vi "Test App Process Error Handler is Used if Configured.vi"(8 "error in (no error)":errorcluster, 11 "Rig Test In":refnum<class "Application Test.lvclass">) -> (0 "error out":errorcluster, 3 "Rig Test Out":refnum<class "Application Test.lvclass">)   [LabVIEW 2020, in "Application Test.lvclass"]
uses:
  Application Test.lvclass
  C:/Program Files (x86)/National Instruments/LabVIEW 2020/vi.lib/Asteme/LUnit/Test Case.lvclass
  Mock Process/Mock Process.lvclass
  C:/Users/anton/Documents/GitHub/Triarc-Framework/source/Framework/Process/Process.lvclass
  Mock Error Handler/Mock Error Handler.lvclass
  C:/Users/anton/Documents/GitHub/Triarc-Framework/source/Framework/Error Handler Interface/Error Handler Interface.lvclass
  Framework/Process/Process.lvclass/Process.ctl
  Framework/Application/Application.lvclass/Application.ctl
  <vilib>/Asteme/LUnit/Test Case.lvclass/Test Case.ctl
  <vilib>/Asteme/LUnit/LUnit Assertion Result.lvclass/LUnit Assertion Result.ctl
  Framework/Process/Protected/Messaging/Enqueue Message.vi
  Framework/Process/Public/Lifecycle/Get Lifecycle State.vi
  Framework/Application/Private/Add Process to Map.vi
  Framework/Process/Protected/SubVIs/Set Context.vi
  Framework/Process/Protected/Messaging/Request Message.vi
  <vilib>/Asteme/LUnit/Palette/Pass.vi
  <vilib>/Asteme/LUnit/Palette/Fail.vi
  <vilib>/Asteme/LUnit/Variant to string.vi
  <vilib>/Asteme/LUnit/Set Assertion Type.vi
  Framework/Process/Private/SubVIs/Wait for finish.vi
  Framework/Process/Private/SubVIs/Set Lifecycle State.vi
  <vilib>/Utility/error.llb/Clear Errors.vi
  Framework/Process/Community/Leave Process Loop.vi
  Framework/Process/Private/SubVIs/Enqueue Request Message.vi
  <vilib>/Asteme/LUnit/Add test result.vi
  <vilib>/Asteme/LUnit/LUnit Write Passed.vi
  <vilib>/Asteme/LUnit/LUnit Get Test Case.vi
  <vilib>/Asteme/LUnit/Assertion Result/LUnit Get Test Name.vi
  <vilib>/Asteme/LUnit/LUnit Write Message.vi
  <vilib>/Asteme/LUnit/LUnit Write Description.vi
  <vilib>/Asteme/LUnit/LUnit Write Assertion Type.vi
  <vilib>/Asteme/LUnit/Read Test Case Name.vi
  Framework/Application/Application.lvclass
  <vilib>/Utility/error.llb/Error Cluster From Error Code.vi
  Framework/Application/Private/Update Context for Owned Processes.vi
  Framework/Process/Private/SubVIs/Wait for Response Message.vi
  <vilib>/Utility/Data Type/Get Type Information.vi
  <vilib>/Utility/LVClass/Get LV Class Name.vi
  Framework/Process/Process.lvclass
  <vilib>/Asteme/LUnit/LUnit Assertion Result.lvclass
  <vilib>/Asteme/LUnit/Test Case.lvclass
  C:/Users/anton/Documents/GitHub/Triarc-Framework/source/Framework/Base/Base.lvclass
  C:/Users/anton/Documents/GitHub/Triarc-Framework/source/Framework/Logging/Logging.lvclass
  C:/Users/anton/Documents/GitHub/Triarc-Framework/source/Framework Test/Mock Process/Mock Process.lvclass
  C:/Users/anton/Documents/GitHub/Triarc-Framework/source/Framework/Helper Loop/Helper Loop.lvclass
  C:/Users/anton/Documents/GitHub/Triarc-Framework/source/Framework/Application/Application.lvclass
  C:/Users/anton/Documents/GitHub/Triarc-Framework/source/Framework Test/Process Test/Process Test.lvclass
  C:/Users/anton/Documents/GitHub/Triarc-Framework/source/Framework Test/Base Class Test/Base Test.lvclass
  C:/Users/anton/Documents/GitHub/Triarc-Framework/source/Framework Test/Application Test/Application Test.lvclass
  C:/Users/anton/Documents/GitHub/Triarc-Framework/source/Framework Test/Mock Error Handler/Mock Error Handler.lvclass
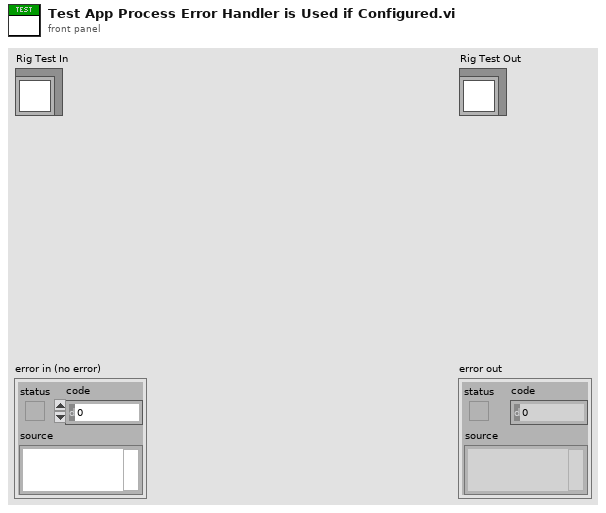
[diagram p1: front panel]
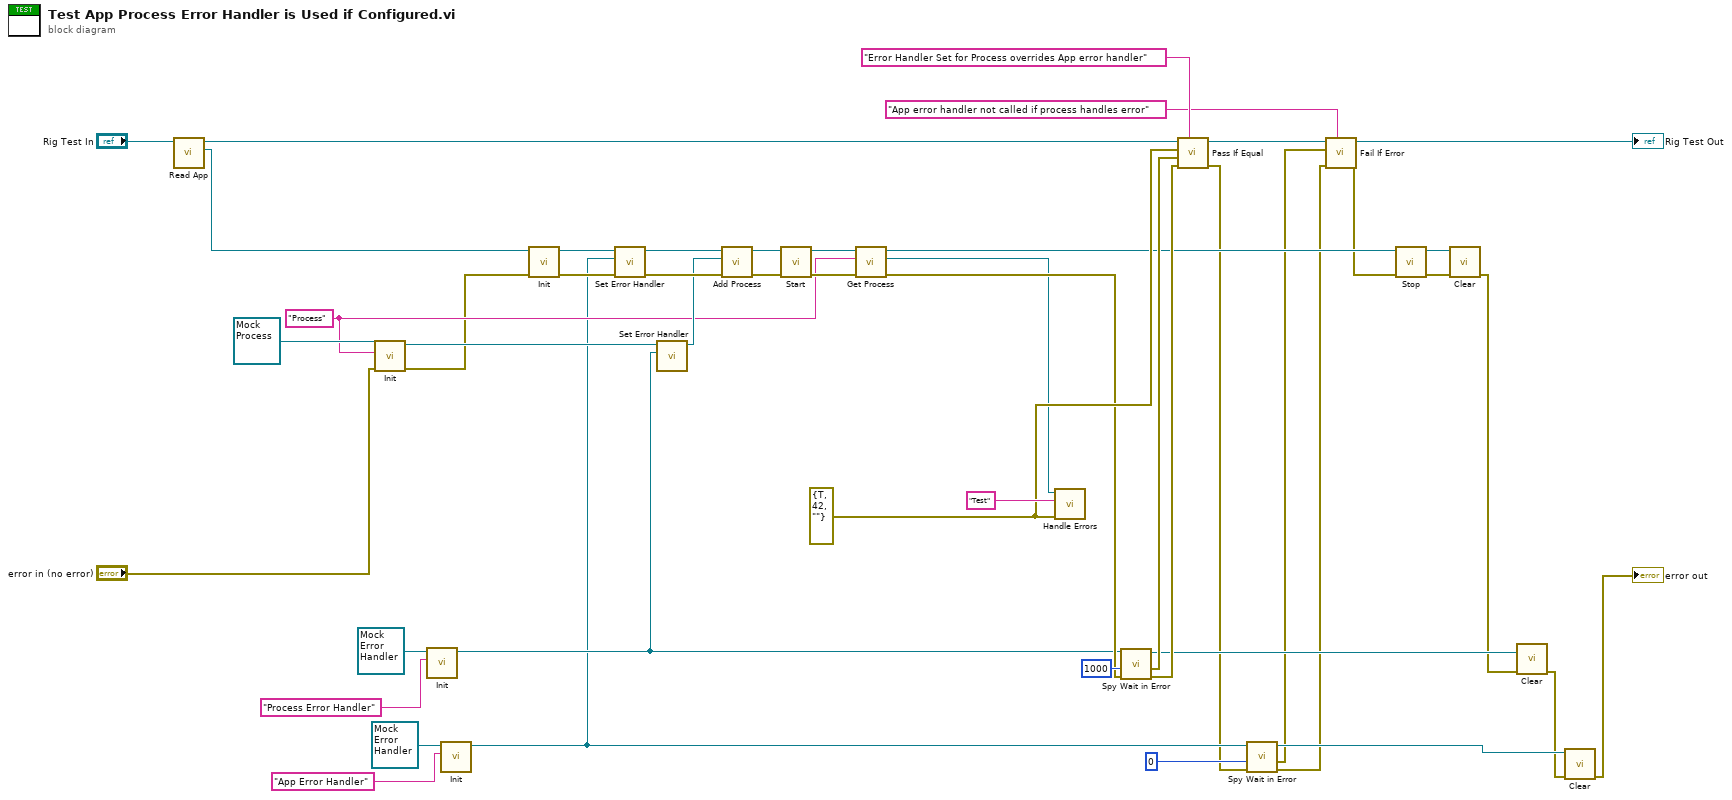
[diagram p0: block diagram]
diagram:
  w21 = "Process" ("Name")
  w40 = errorcluster {"status"=TRUE, "code"=42, "source"=""} ("error in (no error)")
  n1 = call "Read App.vi"("Application Test In"="Rig Test In") -> ("App out"=w31:refnum<class "Application.lvclass">, "Application Test Out"=w44:refnum<class "Application Test.lvclass">)  [unwired: 8 in, 1 out]
  n2 = call-dynamic "Init.vi"("error in (no error)"="error in (no error)", "Name"=w21, "Mock Process In"=refnum<class "Mock Process.lvclass"> refnum ("Mock Process.lvclass")) -> ("error out"=w7:errorcluster, "Mock Process Out"=w19:refnum<class "Mock Process.lvclass">)  [unwired: 7 in]
  n3 = call-dynamic "Init.vi"("Name"="Process Error Handler", "Mock Error Handler In"=refnum<class "Mock Error Handler.lvclass"> refnum ("Mock Error Handler.lvclass")) -> ("Mock Error Handler Out"=w16:refnum<class "Mock Error Handler.lvclass">)  [unwired: 8 in, 1 out]
  n4 = call-dynamic "Init.vi"("Name"="App Error Handler", "Mock Error Handler In"=refnum<class "Mock Error Handler.lvclass"> refnum ("Mock Error Handler.lvclass")) -> ("Mock Error Handler Out"=w14:refnum<class "Mock Error Handler.lvclass">)  [unwired: 8 in, 1 out]
  n5 = call-dynamic "Init.vi"("error in (no error)"=w7, "Process In"=w31) -> ("error out"=w29:errorcluster, "Process Out"=w25:refnum<class "Application.lvclass">)  [unwired: 8 in]
  n6 = call "Set Error Handler.vi"("error in (no error)"=w29, "Error Handler"=w14, "Process In"=w25) -> ("error out"=w26:errorcluster, "Process Out"=w24:refnum<class "Application.lvclass">)  [unwired: 7 in]
  n7 = call "Set Error Handler.vi"("Error Handler"=w16, "Process In"=w19) -> ("Process Out"=w23:refnum<class "Mock Process.lvclass">)  [unwired: 8 in, 1 out]
  n8 = call "Add Process.vi"("error in (no error)"=w26, "Process"=w23, "Rig In"=w24) -> ("error out"=w36:errorcluster, "Rig Out"=w33:refnum<class "Application.lvclass">)  [unwired: 7 in]
  n9 = call "Start.vi"("error in (no error)"=w36, "Process In"=w33) -> ("error out"=w34:errorcluster, "Process Out"=w32:refnum<class "Application.lvclass">)  [unwired: 8 in]
  n10 = call "Get Process.vi"("error in (no error)"=w34, "Process Name"=w21, "Rig In"=w32) -> ("error out"=w27:errorcluster, "App Process"=w20:refnum<class "Process.lvclass">, "Rig Out"=w28:refnum<class "Application.lvclass">)  [unwired: 6 in]
  n11 = call-dynamic "Handle Errors.vi"("error in (no error)"=w40, "Location"="Test", "Process In"=w20) -> ()  [unwired: 7 in, 2 out]
  n12 = call "Spy Wait in Error.vi"("error in (no error)"=w27, "timeout in ms (-1)"=1000, "Mock Error Handler In"=w16) -> ("error out"=w38:errorcluster, "Errors"=w39:errorcluster, "Mock Error Handler Out"=w13:refnum<class "Mock Error Handler.lvclass">)  [unwired: 4 in, 2 out]
  n13 = call <vilib>:"Pass If Equal.vi"("Description"="Error Handler Set for Process overrides App error handler", "error in (no error)"=w38, "Actual"=w39, "Expected"=w40, "Test Case In"=w44) -> ("error out"=w11:errorcluster, "Test Case Out"=w5:refnum<class "Application Test.lvclass">)  [unwired: 5 in]
  n14 = call "Spy Wait in Error.vi"("error in (no error)"=w11, "timeout in ms (-1)"=0, "Mock Error Handler In"=w14) -> ("error out"=w3:errorcluster, "Errors"=w2:errorcluster, "Mock Error Handler Out"=w12:refnum<class "Mock Error Handler.lvclass">)  [unwired: 4 in, 2 out]
  n15 = call <vilib>:"Fail If Error.vi"("Description"="App error handler not called if process handles error", "error in (no error)"=w3, "Assert error"=w2, "Test Case In"=w5) -> ("error out"=w6:errorcluster, "Test Case Out"=→"Rig Test Out":refnum<class "Application Test.lvclass">)  [unwired: 6 in]
  n16 = call "Stop.vi"("error in (no error)"=w6, "Process In"=w28) -> ("error out"=w30:errorcluster, "Process Out"=w35:refnum<class "Application.lvclass">)  [unwired: 7 in, 1 out]
  n17 = call-dynamic "Clear.vi"("error in (no error)"=w30, "Application In"=w35) -> ("error out"=w9:errorcluster)  [unwired: 9 in]
  n18 = call-dynamic "Clear.vi"("error in (no error)"=w9, "Mock Process In"=w13) -> ("error out"=w10:errorcluster)  [unwired: 9 in]
  n19 = call-dynamic "Clear.vi"("error in (no error)"=w10, "Mock Process In"=w12) -> ("error out"=→"error out":errorcluster)  [unwired: 9 in]
